vi "ShowHexValues.vi"(1 "String":string) -> (0 "String 2":string)   [LabVIEW 2014]
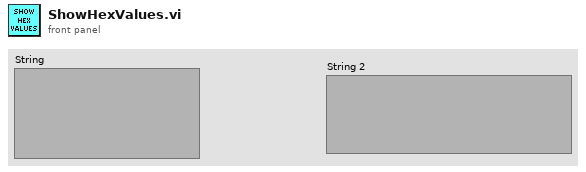
[diagram p1: front panel]
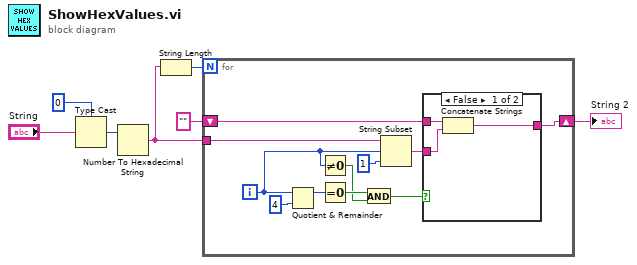
[diagram p0: block diagram]
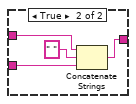
[diagram p2: hidden frame]
diagram:
  n1 = Type Cast(type=0, x="String") -> (*(type *) &x=w5:i32)
  n2 = Number To Hexadecimal String(2:w5) -> (0:w3:string)  [unwired: 1 in]
  n3 = String Length(string=w3) -> (length=w4:i32)
  n4 = for {
    N: w4 -> [_]
    tunnel: w3 -> [w18]
    shift-right: [w13] -> w1
    shift-left: "" -> [w12]
    i -> [w11]
    n5 = Quotient & Remainder(x=w11, y=4) -> (x-y*floor(x/y)=w15:i32)  [unwired: 1 out]
    n6 = Not Equal To 0?(x=w11) -> (x != 0?=w9:bool)
    n7 = Equal To 0?(x=w15) -> (x = 0?=w10:bool)
    n8 = And(x=w10, y=w9) -> (x .and. y?=w8:bool)
    n9 = String Subset(string=w18, offset (0)=w11, length (rest)=1 ("length (rest)")) -> (substring=w14:string)
    n10 = case shown="False" w8 {
      tunnel: w14 -> [w21 w25]
      tunnel: [w19 w23] -> w13
      tunnel: w12 -> [w20 w22]
      frame False {
        n11 = Concatenate Strings(w20, w21) -> (w19:string)
      }
      frame True {
        n12 = Concatenate Strings(w22, " " ("string"), w25) -> (w23:string)
      }
    }
  }
  "String 2" <- w1
